vi "DQMH Get Fully Delimited Instance Name from Module Name.vi"(8 "error in":errorcluster, 10 "Module Name":string, 11 "Module Path":path) -> (0 "error out":errorcluster, 2 "Main VI (Full Delimited Name)":string)   [LabVIEW 2022 SP3, in "hse-dqmh.lvlib"]
doc: "Parses the fully delimited VI name from the module path and the module name. For cloneables, the clone ID is appended to the VI name.\n\n____\nHAMPEL SOFTWARE ENGINEERING v3.8.0 (2023-12-18 14:41)"
uses:
  hse-dqmh.lvlib
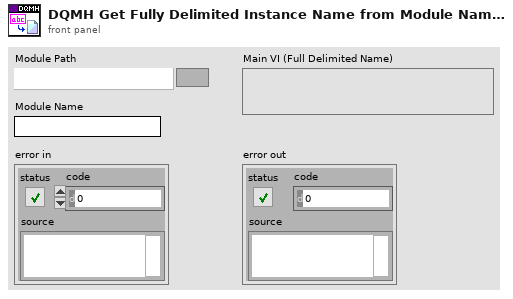
[diagram p1: front panel]
types:
  T1 = typedef "hse-dqmh.lvlib/Module Types.ctl" = enum16{"Singleton", "Cloneable"}
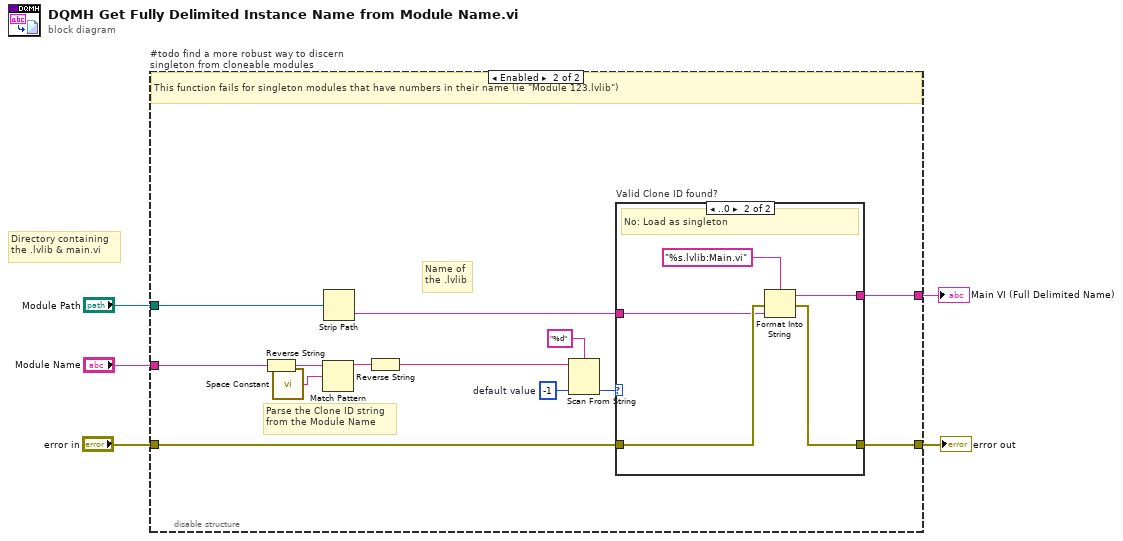
[diagram p0: block diagram]
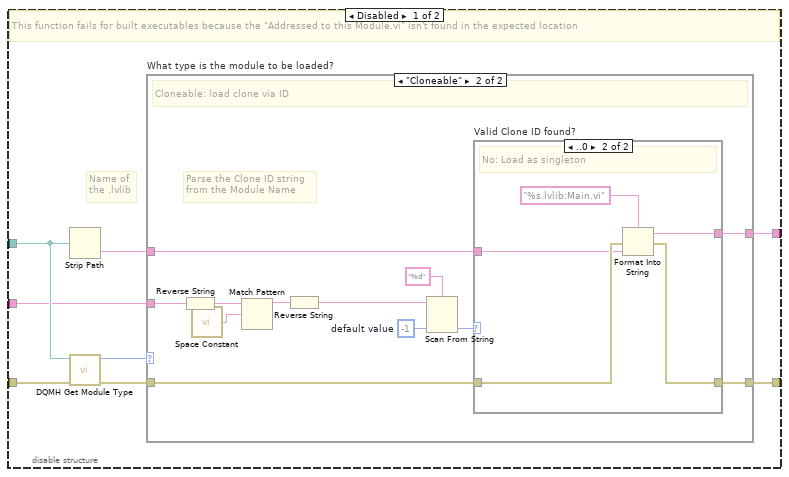
[diagram p2: hidden frame]
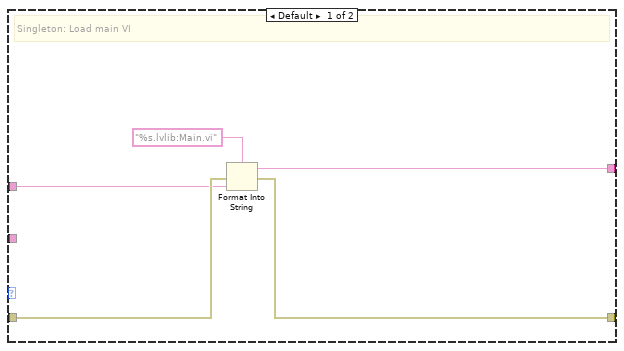
[diagram p3: hidden frame]
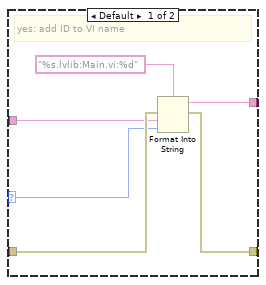
[diagram p4: hidden frame]
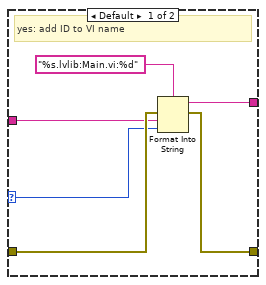
[diagram p5: hidden frame]
diagram:
  # "Directory containing\nthe .lvlib & main.vi"
  n1 = disable-structure "#todo find a more robust way to discern singleton from cloneable modules" shown="Enabled" {
    disable-tunnel: [w13 w54] -> w5
    disable-tunnel: "Module Path" -> [w11 w52]
    disable-tunnel: "error in" -> [w10 w51]
    disable-tunnel: "Module Name" -> [w8 w50]
    disable-tunnel: [w7 w49] -> w1
    frame Disabled {
      # "Name of\nthe .lvlib"
      # "This function fails for built executables because the \"Addressed to this Module.vi\" isn't found in the expected location"
      n2 = Strip Path(path=w11) -> (name=w12:string)  [unwired: 1 out]
      n3 = call "DQMH Get Module Type.vi"("error in"=w10, "Module Path"=w11) -> ("error out"=w9:errorcluster, "Module Types"=w6:T1)  [unwired: 8 in]
      n4 = case "What type is the module to be loaded?" shown="\"Cloneable\"" w6 {
        tunnel: [w16 w29] -> w13
        tunnel: w12 -> [w15 w28]
        tunnel: w8 -> [_ w22]
        tunnel: w9 -> [w18 w30]
        tunnel: [w14 w21] -> w7
        frame Default {
          # "Singleton: Load main VI"
          n5 = Format Into String(format string="%s.lvlib:Main.vi" ("name or relative path"), error in=w18, w15) -> (resulting string=w16:string, error out=w14:errorcluster)  [unwired: 1 in]
        }
        frame "Cloneable" {
          w27 = -1  # default value
          # "Parse the Clone ID string\nfrom the Module Name"
          # "Cloneable: load clone via ID"
          n6 = Reverse String(1:w22) -> (0:w23:string)
          n7 = call <vilib>:"Space Constant.vi"() -> ("String"=w24:string)
          n8 = Match Pattern(string=w23, regular expression=w24) -> (before substring=w25:string)  [unwired: 1 in, 3 out]
          n9 = Reverse String(1:w25) -> (0:w20:string)
          n10 = Scan From String(format string="%d", input string=w20, default 1=w27) -> (output 1=w19:i32)  [unwired: 2 in, 3 out]
          n11 = case "Valid Clone ID found?" shown="..0" w19 {
            selector: w19 -> [w32 _]
            tunnel: w30 -> [w36 w41]
            tunnel: [w35 w40] -> w29
            tunnel: w28 -> [w33 w38]
            tunnel: [w31 w37] -> w21
            frame Default {
              # "yes: add ID to VI name"
              n12 = Format Into String(format string="%s.lvlib:Main.vi:%d" ("name or relative path"), error in=w36, w33, w32) -> (resulting string=w35:string, error out=w31:errorcluster)  [unwired: 1 in]
            }
            frame ..0 {
              # "No: Load as singleton"
              n13 = Format Into String(format string="%s.lvlib:Main.vi" ("name or relative path"), error in=w41, w38) -> (resulting string=w40:string, error out=w37:errorcluster)  [unwired: 1 in]
            }
          }
        }
      }
    }
    frame Enabled {
      w48 = -1  # default value
      # "Parse the Clone ID string\nfrom the Module Name"
      # "Name of\nthe .lvlib"
      # "This function fails for singleton modules that have numbers in their name (ie \"Module 123.lvlib\")"
      n14 = Reverse String(1:w50) -> (0:w44:string)
      n15 = call <vilib>:"Space Constant.vi"() -> ("String"=w45:string)
      n16 = Match Pattern(string=w44, regular expression=w45) -> (before substring=w46:string)  [unwired: 1 in, 3 out]
      n17 = Strip Path(path=w52) -> (name=w53:string)  [unwired: 1 out]
      n18 = Reverse String(1:w46) -> (0:w43:string)
      n19 = Scan From String(format string="%d", input string=w43, default 1=w48) -> (output 1=w42:i32)  [unwired: 2 in, 3 out]
      n20 = case "Valid Clone ID found?" shown="..0" w42 {
        selector: w42 -> [w56 _]
        tunnel: w51 -> [w60 w65]
        tunnel: [w59 w64] -> w54
        tunnel: w53 -> [w57 w62]
        tunnel: [w55 w61] -> w49
        frame Default {
          # "yes: add ID to VI name"
          n21 = Format Into String(format string="%s.lvlib:Main.vi:%d" ("name or relative path"), error in=w60, w57, w56) -> (resulting string=w59:string, error out=w55:errorcluster)  [unwired: 1 in]
        }
        frame ..0 {
          # "No: Load as singleton"
          n22 = Format Into String(format string="%s.lvlib:Main.vi" ("name or relative path"), error in=w65, w62) -> (resulting string=w64:string, error out=w61:errorcluster)  [unwired: 1 in]
        }
      }
    }
  }
  "Main VI (Full Delimited Name)" <- w5
  "error out" <- w1
